vi "outputDebugString.vi"(11 "arg1":string) -> ()   [LabVIEW 2018]
uses:
  C:/Windows/System32/kernel32.dll
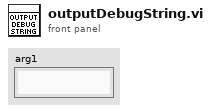
[diagram p1: front panel]
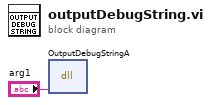
[diagram p0: block diagram]
diagram:
  n1 = dll-call lib="C:/Windows/System32/kernel32.dll" fn="OutputDebugStringA"("arg1"="arg1") -> ()  [unwired: 5 in, 2 out]
